vi "knob(v2021).vi"() -> ()   [LabVIEW 2021]
panel:
  out "Numeric":dbl
  in  "VISA resource name":refnum<visa-resource-name>
  in  "Knob":dbl(knob) scale=0.0..100.0
  in  "stop":bool
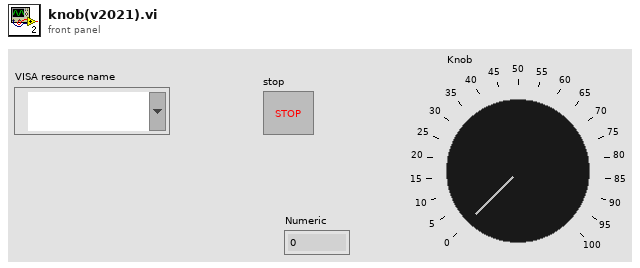
[diagram p1: front panel]
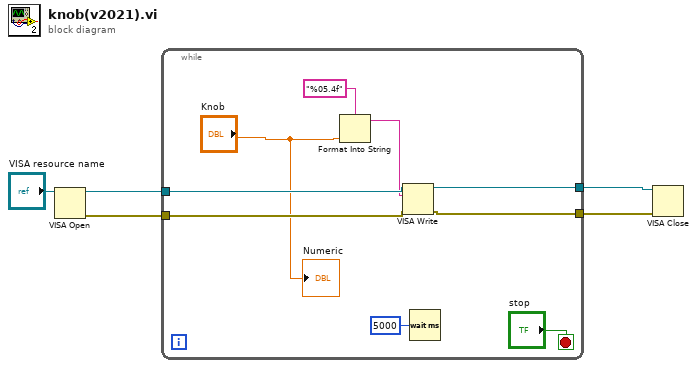
[diagram p0: block diagram]
diagram:
  n1 = VISA Open(VISA resource name="VISA resource name") -> (VISA resource name=w5:refnum<visa-resource-name>, error out=w4:errorcluster)  [unwired: 4 in]
  n2 = while {
    tunnel: w5 -> [w12]
    tunnel: w4 -> [w11]
    tunnel: [w10] -> w3
    tunnel: [w9] -> w2
    stop <- "stop" stop-if-true
    n3 = Format Into String(format string="%05.4f", "Knob") -> (resulting string=w8:string)  [unwired: 2 in, 1 out]
    n4 = VISA Write(VISA resource name=w12, write buffer=w8, error in (no error)=w11) -> (VISA resource name out=w10:refnum<visa-resource-name>, error out=w9:errorcluster)  [unwired: 1 out]
    n5 = Wait (ms)(milliseconds to wait=u32 5000) -> ()  [unwired: 1 out]
    "Numeric" <- "Knob"
  }
  n6 = VISA Close(VISA resource name=w3, error in (no error)=w2) -> ()  [unwired: 1 out]
